vi "Get Attribute STRING.vi"(8 "error in":errorcluster, 10 "Attribute":string, 11 "IConfigurable in":refnum<class "IConfigurable.lvclass">) -> (0 "error out":errorcluster, 2 "Value":string, 3 "IConfigurable out":refnum<class "IConfigurable.lvclass">)   [LabVIEW 2024, in "IConfigurable.lvclass"]
uses:
  IConfigurable.lvclass
  IConfiguration/IConfiguration.lvclass
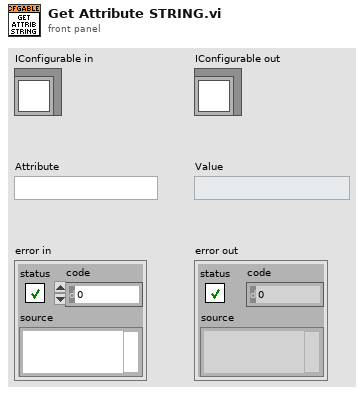
[diagram p1: front panel]
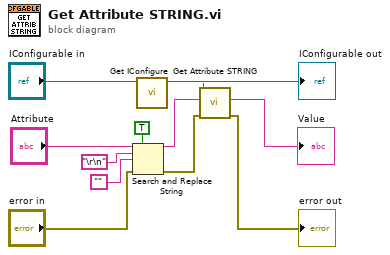
[diagram p0: block diagram]
diagram:
  n1 = Search and Replace String(replace all?=TRUE ("replace all? (F)"), input string="Attribute", search string="\r\n", replace string="", error in="error in") -> (result string=w6:string, error out=w2:errorcluster)  [unwired: 3 in, 2 out]
  n2 = call-dynamic "Get IConfigure.vi"("IConfigurable in"="IConfigurable in") -> ("IConfigure"=w10:refnum<class "IConfigure.lvclass">, "IConfigurable out"=→"IConfigurable out":refnum<class "IConfigurable.lvclass">)  [unwired: 8 in, 1 out]
  n3 = call-dynamic "Get Attribute STRING.vi"("error in"=w2, "Attribute"=w6, "IConfiguration in"=w10) -> ("error out"=→"error out":errorcluster, "Value"=→"Value":string)  [unwired: 6 in, 1 out]
